vi "Synth Real Cfg to Integer.vi"(0 "Frequency(kHz)":dbl=100.0 format="%#.10f", 1 "Phase(Degrees)":dbl=90.0, 2 "IF (Hz)":dbl format="%.2f") -> (5 "Phase word":u8 format="%08b", 6 "f-word":u32, 7 "IF":u32)   [LabVIEW 2016]
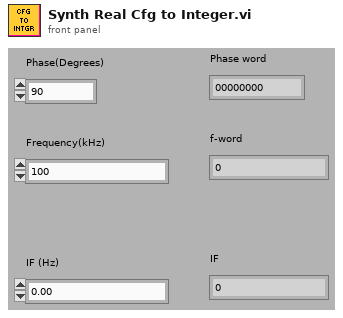
[diagram p1: front panel]
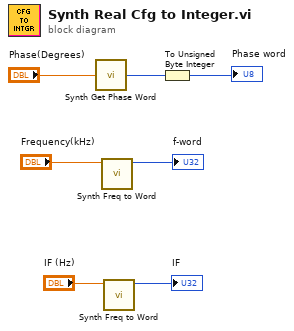
[diagram p0: block diagram]
diagram:
  n1 = call "Synth Get Phase Word.vi"("Phase"="Phase(Degrees)") -> ("Phase Byte"=w5:u8)
  n2 = call "Synth Freq to Word.vi"("Frequency (Hz)"="Frequency(kHz)") -> ("f-word out"=→"f-word":u32)  [unwired: 8 in, 2 out]
  n3 = call "Synth Freq to Word.vi"("Frequency (Hz)"="IF (Hz)") -> ("f-word out"=→"IF":u32)  [unwired: 8 in, 2 out]
  n4 = To Unsigned Byte Integer(number=w5) -> (unsigned 8bit integer=→"Phase word":u8)
